vi "MUX.vi"(0 "Start":bool, 1 "LS1":bool, 2 "LS2":bool, 3 "LS3":bool, 4 "LS4":bool, 5 "LS5":bool, 6 "Pause":bool, 7 "Stop":bool, 8 "UP":bool, 10 "DOWN":bool, 12 "EXTEND":bool, 14 "BACK":bool) -> (15 "Enum":T1)   [LabVIEW 2017]
uses:
  state_D.ctl
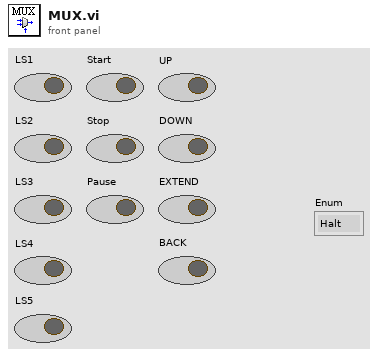
[diagram p1: front panel]
types:
  T1 = typedef "state_D.ctl" = enum16{"Halt", "Start", "LS1", "LS2", "LS3", "LS4", "LS5", "UP", "DOWN", "EXTEND", "BACK", "Stop", "Pause"}
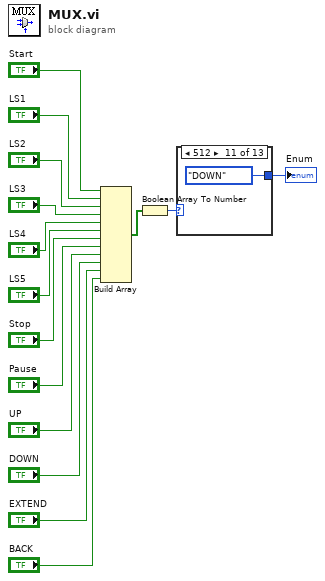
[diagram p0: block diagram]
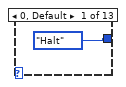
[diagram p2: hidden frame]
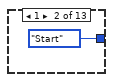
[diagram p3: hidden frame]
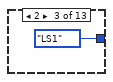
[diagram p4: hidden frame]
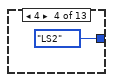
[diagram p5: hidden frame]
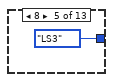
[diagram p6: hidden frame]
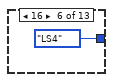
[diagram p7: hidden frame]
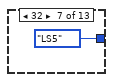
[diagram p8: hidden frame]
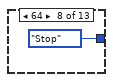
[diagram p9: hidden frame]
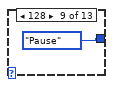
[diagram p10: hidden frame]
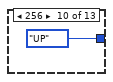
[diagram p11: hidden frame]
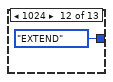
[diagram p12: hidden frame]
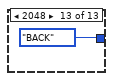
[diagram p13: hidden frame]
diagram:
  n1 = Build Array("Start", "LS1", "LS2", "LS3", "LS4", "LS5", "Stop", "Pause", "UP", "DOWN", "EXTEND", "BACK") -> (w14:bool[])
  n2 = Boolean Array To Number(Boolean array=w14) -> (number=w15:u32)
  n3 = case shown="512" w15 {
    tunnel: [state_D."Halt" ("Enum") state_D."Start" ("Enum") state_D."LS1" ("Enum") state_D."LS2" ("Enum") state_D."LS3" ("Enum") state_D."LS4" ("Enum") state_D."LS5" ("Enum") state_D."Stop" ("Enum") state_D."Pause" ("Enum") state_D."UP" ("Enum") state_D."DOWN" ("Enum") state_D."EXTEND" ("Enum") state_D."BACK" ("Enum")] -> w13
    frame 0, Default {
    }
    frame 1 {
    }
    frame 2 {
    }
    frame 4 {
    }
    frame 8 {
    }
    frame 16 {
    }
    frame 32 {
    }
    frame 64 {
    }
    frame 128 {
    }
    frame 256 {
    }
    frame 512 {
    }
    frame 1024 {
    }
    frame 2048 {
    }
  }
  "Enum" <- w13
